vi "Framework Listener Sobot.vi"() -> ()   [LabVIEW 2017]
uses:
  TypeDefinitions/TCP Cluster.ctl
  TypeDefinitions/TCP Commands.ctl
  <vilib>/Instr/_visa.llb/VISA Configure Serial Port (Instr).vi
panel:
  in  "VISA resource name":refnum<visa-resource-name>
  out "Received Message":string
  out "Receive":T1={"Datatype"=enum."Message", "String"="Send to sobot"}
  out "Send":T1={"Datatype"=enum."Message", "String"="Send to sobot"}
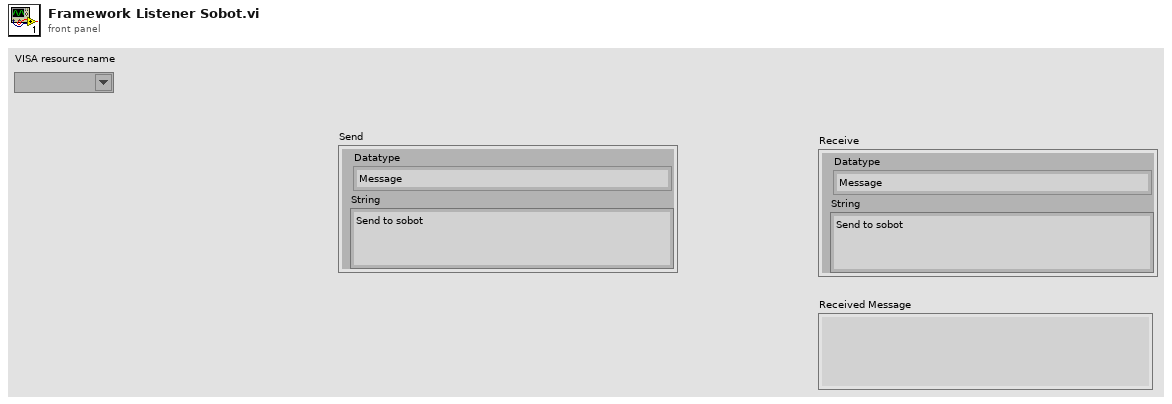
[diagram p1: front panel]
types:
  T1 = typedef "TCP Cluster.ctl" = cluster{"Datatype":T2, "String":string}
  T2 = typedef "TCP Commands.ctl" = enum16{"Timeout", "Log", "Message", "ManualDrive", "Stop", "Command"}
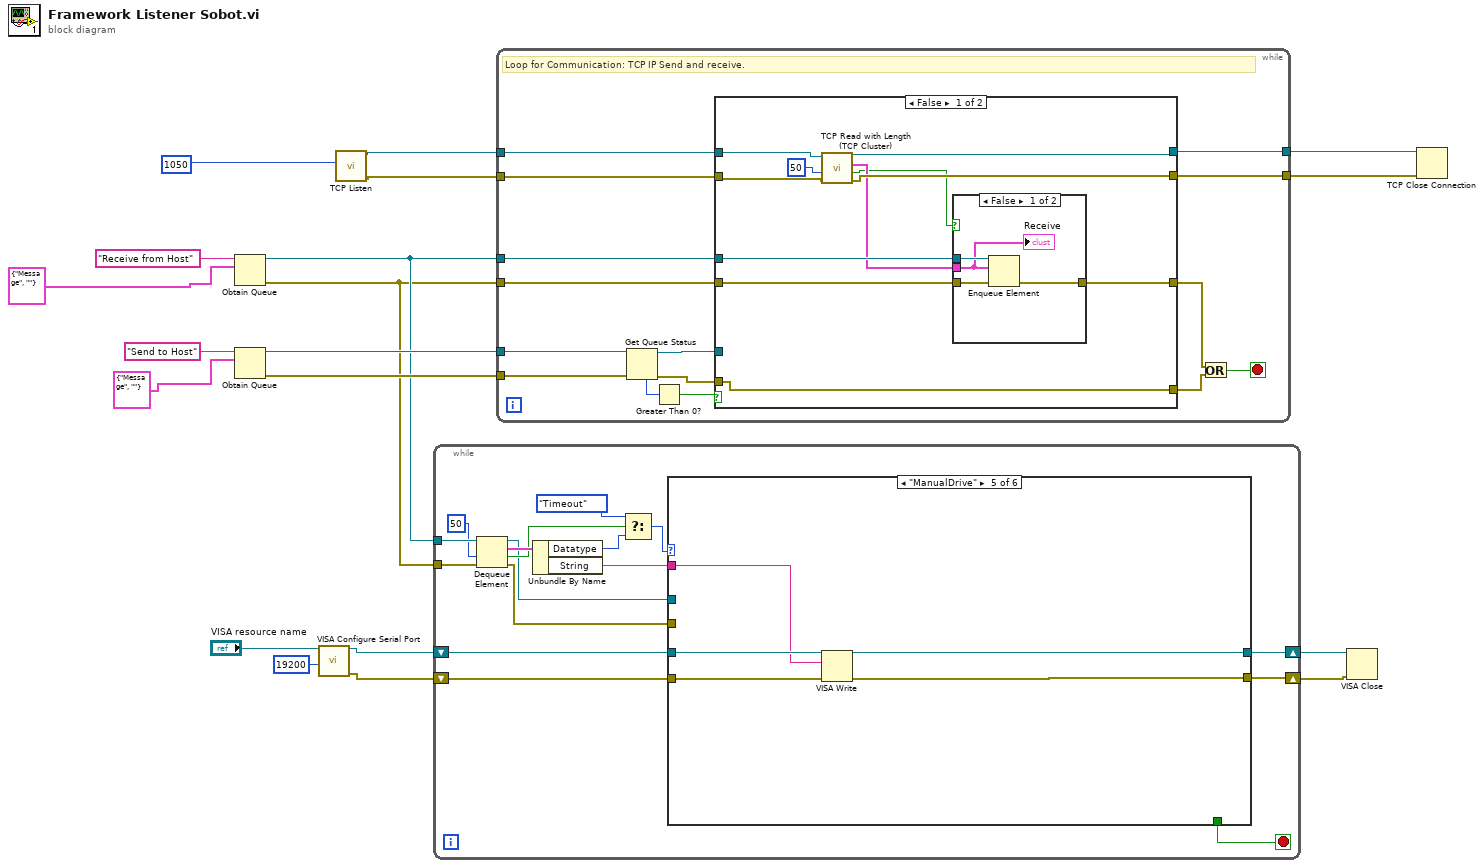
[diagram p0: block diagram]
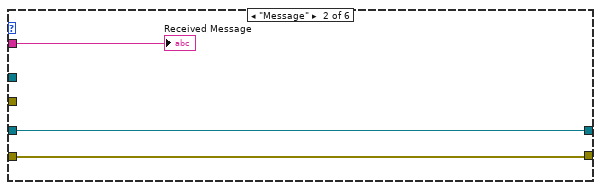
[diagram p3: hidden frame]
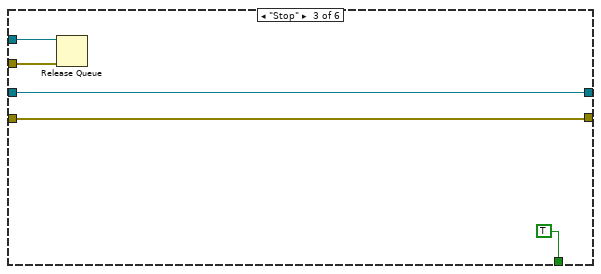
[diagram p4: hidden frame]
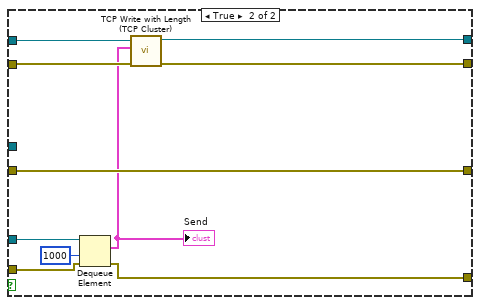
[diagram p8: hidden frame]
diagram:
  n1 = Obtain Queue(name (unnamed)="Receive from Host", element data type=T1 {"Datatype"=enum."Message", "String"=""}) -> (queue out=w8:refnum<queue>, error out=w1:errorcluster)  [unwired: 3 in, 1 out]
  n2 = Obtain Queue(name (unnamed)="Send to Host", element data type=T1 {"Datatype"=enum."Message", "String"=""}) -> (queue out=w13:refnum<queue>, error out=w12:errorcluster)  [unwired: 3 in, 1 out]
  n3 = call-poly "VISA Configure Serial Port"("VISA resource name"="VISA resource name", "baud rate (9600)"=u32 19200) -> ("VISA resource name out"=w7:refnum<visa-resource-name>, "error out"=w6:errorcluster)  [unwired: 12 in]
  n4 = call <vilib>:"TCP Listen.vi"("port"=u16 1050 ("remote port or service name")) -> ("error out"=w10:errorcluster, "connection ID"=w11:refnum<k5>)  [unwired: 6 in, 3 out]
  n5 = while {
    tunnel: w8 -> [w35]
    shift-right: [w31] -> w3
    shift-left: w7 -> [w29]
    shift-right: [w32] -> w2
    shift-left: w6 -> [w30]
    tunnel: w1 -> [w26]
    stop <- w27 stop-if-true
    n6 = Dequeue Element(queue=w35, timeout in ms (-1)=50, error in (no error)=w26) -> (queue out=w21:refnum<queue>, element=w34:T1, timed out?=w24:bool, error out=w20:errorcluster)
    n7 = Unbundle By Name(w34) -> ("Datatype"=w23:T2, "String"=w33:string)
    n8 = Select(t=TCP_Commands."Timeout", s=w24, f=w23) -> (s? t:f=w25:T2)
    n9 = case shown="\"ManualDrive\"" w25 {
      tunnel: w33 -> [_ w40 _ _ w48 _]
      tunnel: [w36 w38 w44 w46 w49 w53] -> w32
      tunnel: [w37 w39 w45 w47 w50 w54] -> w31
      tunnel: w30 -> [w36 w38 w44 w46 w51 w53]
      tunnel: w29 -> [w37 w39 w45 w47 w52 w54]
      tunnel: [_ _ TRUE _ _ _] -> w27
      tunnel: w21 -> [_ _ w42 _ _ _]
      tunnel: w20 -> [_ _ w41 _ _ _]
      frame "Log" {
        # "Datenlogging"
      }
      frame "Message" {
        "Received Message" <- w40
      }
      frame "Stop" {
        n10 = Release Queue(queue=w42, error in (no error)=w41) -> ()  [unwired: 1 in, 3 out]
      }
      frame "Command" {
      }
      frame "ManualDrive" {
        n11 = VISA Write(VISA resource name=w52, write buffer=w48, error in (no error)=w51) -> (VISA resource name out=w50:refnum<visa-resource-name>, error out=w49:errorcluster)  [unwired: 1 out]
      }
      frame "Timeout", Default {
      }
    }
  }
  n12 = while {
    tunnel: w13 -> [w69]
    tunnel: w12 -> [w67]
    tunnel: w11 -> [w63]
    tunnel: w10 -> [w62]
    tunnel: [w61] -> w18
    tunnel: [w60] -> w17
    tunnel: w8 -> [w59]
    tunnel: w1 -> [w58]
    stop <- w55 stop-if-true
    # "Loop for Communication: TCP IP Send and receive."
    n13 = Get Queue Status(queue=w69, error in (no error)=w67) -> (queue out=w68:refnum<queue>, error out=w66:errorcluster, # elements in queue=w65:i32)  [unwired: 1 in, 5 out]
    n14 = Greater Than 0?(x=w65) -> (x > 0?=w64:bool)
    n15 = case shown="False" w64 {
      tunnel: [w80 w95] -> w56
      tunnel: w68 -> [_ w93]
      tunnel: w66 -> [w80 w92]
      tunnel: w63 -> [w76 w90]
      tunnel: w62 -> [w75 w89]
      tunnel: [w73 w88] -> w60
      tunnel: [w72 w87] -> w61
      tunnel: w59 -> [w79 _]
      tunnel: w58 -> [w78 w91]
      tunnel: [w77 w91] -> w57
      frame False {
        n16 = call "TCP Read with Length (TCP Cluster).vi"("error in (no error)"=w75, "Timeout"=50, "connection ID"=w76) -> ("error out"=w73:errorcluster, "Timeout?"=w70:bool, "TCP Cluster"=w71:T1, "connection ID out"=w72:refnum<k5>)  [unwired: 5 in]
        n17 = case shown="False" w70 {
          tunnel: w79 -> [w84 _]
          tunnel: w78 -> [w83 w85]
          tunnel: w71 -> [w81 _]
          tunnel: [w82 w85] -> w77
          frame False {
            n18 = Enqueue Element(queue=w84, element=w81, error in (no error)=w83) -> (error out=w82:errorcluster)  [unwired: 1 in, 2 out]
            "Receive" <- w81
          }
          frame True {
          }
        }
      }
      frame True {
        n19 = Dequeue Element(queue=w93, timeout in ms (-1)=1000, error in (no error)=w92) -> (element=w86:T1, error out=w95:errorcluster)  [unwired: 2 out]
        "Send" <- w86
        n20 = call "TCP Write with Length (TCP Cluster).vi"("error in (no error)"=w89, 10:w86, "connection ID"=w90) -> ("error out"=w88:errorcluster, "connection ID out"=w87:refnum<k5>)  [unwired: 7 in]
      }
    }
    n21 = Or(x=w57, y=w56) -> (x .or. y?=w55:bool)
  }
  n22 = VISA Close(VISA resource name=w3, error in (no error)=w2) -> ()  [unwired: 1 out]
  n23 = TCP Close Connection(connection ID=w18, error in (no error)=w17) -> ()  [unwired: 1 in, 2 out]
